vi "Parameters File Handler.vi"(7 "parameters path ctl ref":refnum<vi>, 8 "error in":errorcluster, 10 "selected parameters file":path caption="path to parameters xml", 11 "configuration files page data":T1 {"custom device ref" format="%.0x"}) -> (0 "error out":errorcluster, 3 "configuration files page data out":T1 {"custom device ref" format="%.0x"})   [LabVIEW 2020, in "Ballard ARINC 429 System Explorer.lvlib" / "Implementation.lvlib"]
uses:
  Implementation.lvlib
  Types/Configuration Files Page Data.ctl
  Types/Path Control.ctl
  Types/Browse Button.ctl
  <vilib>/NI VeriStand/Custom Device API/Custom Device Item Ref.ctl
  Import/ARINC 429 Import.lvlib
  Scripting/Ballard/Ballard ARINC 429 Scripting.lvlib
  <vilib>/NI VeriStand/Custom Device API/Custom Device API.lvlib
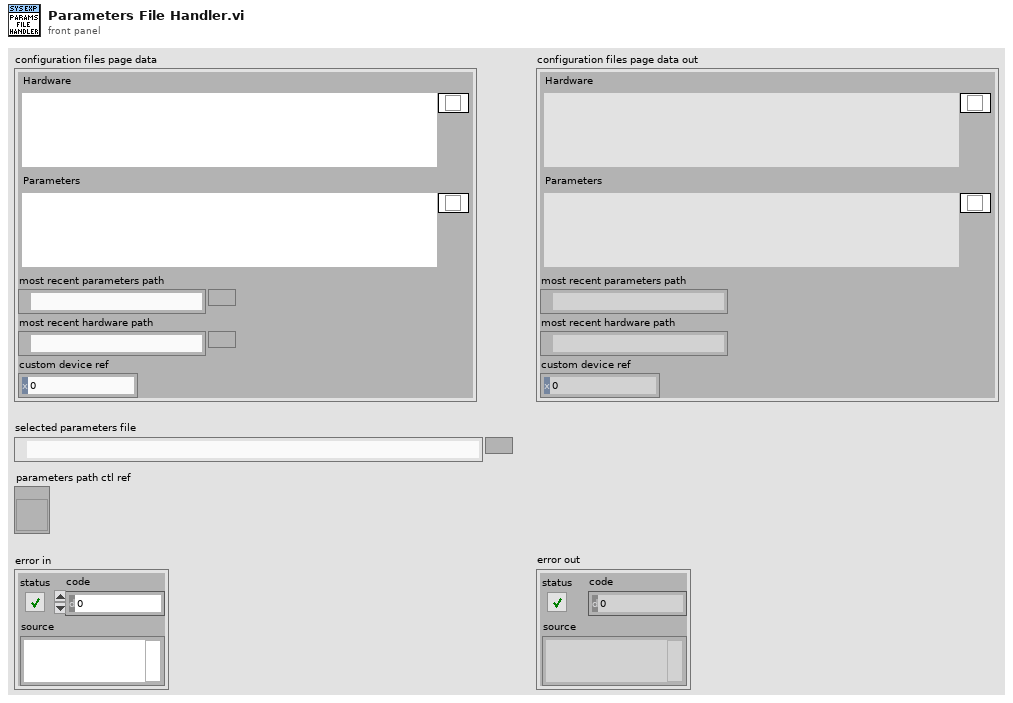
[diagram p1: front panel]
types:
  T1 = typedef "Ballard ARINC 429 System Explorer.lvlib/Implementation.lvlib/Configuration Files Page Data.ctl" = cluster{"Hardware":T2, "Parameters":T2, "most recent parameters path":path, "most recent hardware path":path, "custom device ref":T4}
  T2 = typedef "Ballard ARINC 429 System Explorer.lvlib/Implementation.lvlib/Path Control.ctl" = cluster{"file path":path, "Browse":T3}
  T3 = typedef "Ballard ARINC 429 System Explorer.lvlib/Implementation.lvlib/Browse Button.ctl" = bool
  T4 = typedef "Custom Device API.lvlib/Custom Device Item Ref.ctl" = u64
  T5 = typedef "VS Channels Definition for All Labels on Hardware Channel.ctl" = cluster{"hardware channel":i32, "labels":T6[]}
  T6 = typedef "VS Channels Definition for Label.ctl" = cluster{"label (Dec)":u32, "parameters":T7[], "SDI value":u8, "SDI enabled":bool, "transfer type":T11}
  T7 = typedef "VS Channel Definition for Parameter.ctl" = cluster{"name":string, "direction":T8, "default value":dbl, "unit":string, "Parameter":T9}
  T8 = typedef "Direction.ctl" = enum16{"Rx", "Tx"}
  T9 = typedef "Parameter Definition.ctl" = cluster{"start index":i32, "size":i32, "encoding":T10, "signed":bool, "scale multiplier":dbl, "scale offset":dbl}
  T10 = typedef "Encoding and Decoding.lvlib/Encoding.ctl" = enum16{"BNR", "BCD", "Discrete"}
  T11 = typedef "Transfer Type.ctl" = enum16{"Scheduled", "Acyclic", "Block", "Strobe"}
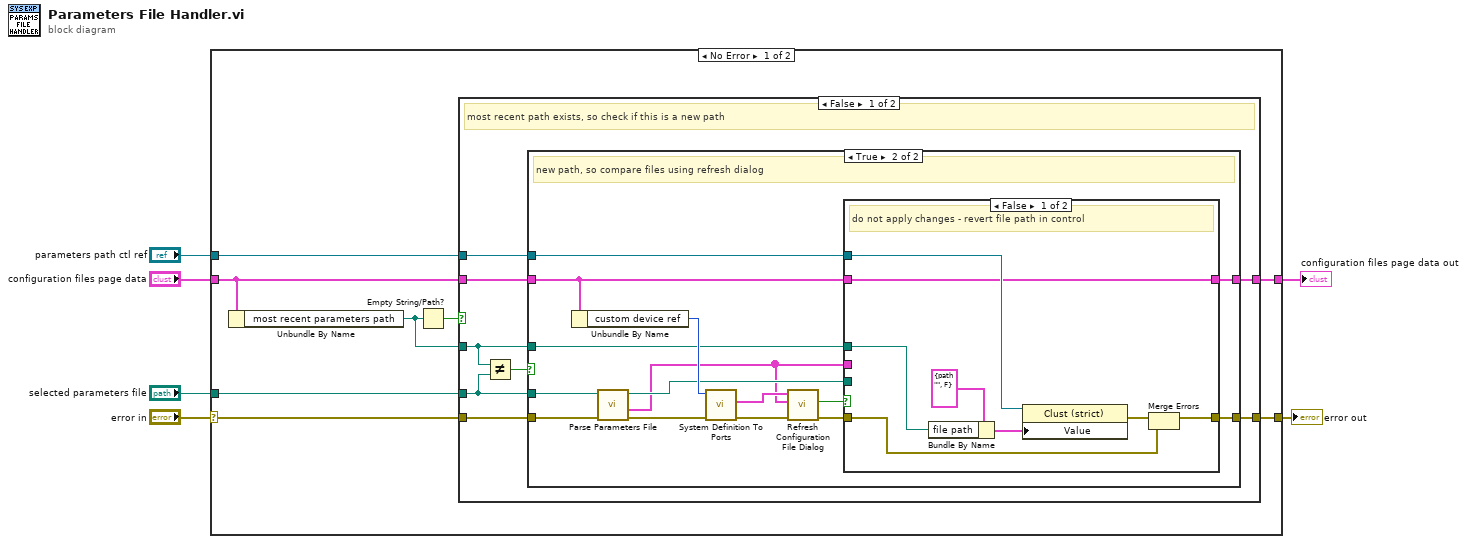
[diagram p0: block diagram]
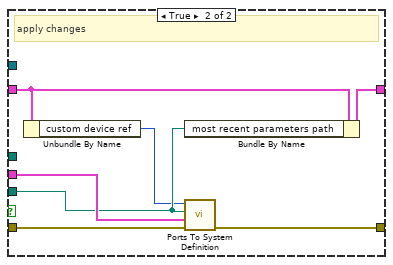
[diagram p3: hidden frame]
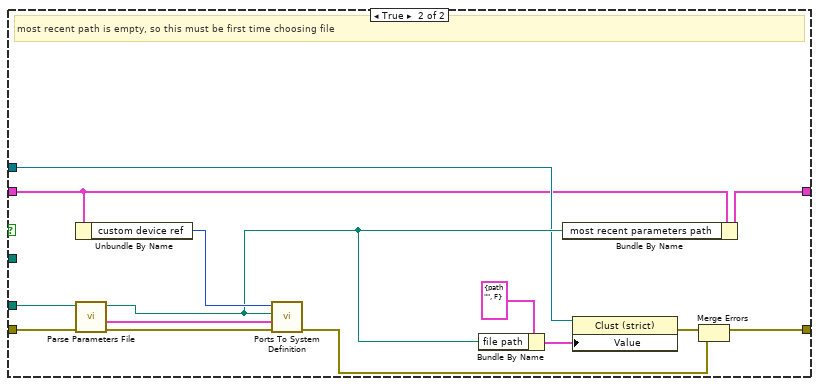
[diagram p4: hidden frame]
diagram:
  n1 = case shown="No Error" "error in" {
    selector: "error in" -> [w14 w70]
    tunnel: [w13 w70] -> w5
    tunnel: "configuration files page data" -> [w11 w69]
    tunnel: [w9 w69] -> w3
    tunnel: "selected parameters file" -> [w12 _]
    tunnel: "parameters path ctl ref" -> [w10 _]
    frame No Error {
      n2 = Unbundle By Name(w11) -> ("most recent parameters path"=w7:path)
      n3 = Empty String/Path?(string/path=w7) -> (empty?=w8:bool)
      n4 = case shown="False" w8 {
        tunnel: w14 -> [w21 w68]
        tunnel: w12 -> [w20 w67]
        tunnel: [w19 w60] -> w13
        tunnel: w7 -> [w18 _]
        tunnel: w11 -> [w17 w56]
        tunnel: w10 -> [w16 w57]
        tunnel: [w15 w55] -> w9
        frame False {
          # "most recent path exists, so check if this is a new path"
          n5 = Not Equal?(x=w18, y=w20) -> (x != y?=w22:bool)
          n6 = case shown="True" w22 {
            tunnel: w21 -> [w24 w39]
            tunnel: w20 -> [_ w28]
            tunnel: [w24 w30] -> w19
            tunnel: w18 -> [_ w29]
            tunnel: w17 -> [w23 w27]
            tunnel: w16 -> [_ w26]
            tunnel: [w23 w25] -> w15
            frame False {
              # "same path, so do nothing"
            }
            frame True {
              # "new path, so compare files using refresh dialog"
              n7 = Unbundle By Name(w27) -> ("custom device ref"=w37:T4)
              n8 = call "Parse Parameters File.vi"("error in"=w39, "path to XML document"=w28) -> ("error out"=w38:errorcluster, "ports"=w31:T5[], "path to XML document out"=w32:path)  [unwired: 7 in]
              n9 = call "System Definition To Ports.vi"("error in"=w38, "custom device ref"=w37) -> ("error out"=w36:errorcluster, "ports"=w35:T5[])  [unwired: 7 in, 1 out]
              n10 = call "Refresh Configuration File Dialog.vi"("error in"=w36, "new ports"=w31, "current ports"=w35) -> ("error out"=w33:errorcluster, "apply changes"=w34:bool)  [unwired: 7 in]
              n11 = case shown="False" w34 {
                tunnel: w33 -> [w42 w54]
                tunnel: w32 -> [_ w52]
                tunnel: w31 -> [_ w53]
                tunnel: [w44 w51] -> w30
                tunnel: w29 -> [w45 _]
                tunnel: w26 -> [w41 _]
                tunnel: w27 -> [w40 w49]
                tunnel: [w40 w50] -> w25
                frame False {
                  # "do not apply changes - revert file path in control"
                  n12 = Bundle By Name(cluster=T2 {"file path"=path "", "Browse"=FALSE} ("Value"), "file path"=w45) -> (w46:T2)
                  n13 = property class="Clust (strict)"(reference=w41, "Value"=w46) -> (error out=w43:errorcluster)  [unwired: 1 in, 1 out]
                  n14 = Merge Errors(w43, w42) -> (w44:errorcluster)
                }
                frame True {
                  # "apply changes"
                  n15 = Unbundle By Name(w49) -> ("custom device ref"=w48:T4)
                  n16 = Bundle By Name(cluster=w49, "most recent parameters path"=w52) -> (w50:T1)
                  n17 = call "Ports To System Definition.vi"("error in"=w54, "ports"=w53, "parameter configuration file path"=w52, "custom device ref"=w48) -> ("error out"=w51:errorcluster)  [unwired: 6 in, 1 out]
                }
              }
            }
          }
        }
        frame True {
          # "most recent path is empty, so this must be first time choosing file"
          n18 = Unbundle By Name(w56) -> ("custom device ref"=w64:T4)
          n19 = call "Parse Parameters File.vi"("error in"=w68, "path to XML document"=w67) -> ("error out"=w66:errorcluster, "ports"=w65:T5[], "path to XML document out"=w58:path)  [unwired: 7 in]
          n20 = call "Ports To System Definition.vi"("error in"=w66, "ports"=w65, "parameter configuration file path"=w58, "custom device ref"=w64) -> ("error out"=w59:errorcluster)  [unwired: 6 in, 1 out]
          n21 = Bundle By Name(cluster=T2 {"file path"=path "", "Browse"=FALSE} ("Value"), "file path"=w58) -> (w63:T2)
          n22 = Bundle By Name(cluster=w56, "most recent parameters path"=w58) -> (w55:T1)
          n23 = property class="Clust (strict)"(reference=w57, "Value"=w63) -> (error out=w61:errorcluster)  [unwired: 1 in, 1 out]
          n24 = Merge Errors(w61, w59) -> (w60:errorcluster)
        }
      }
    }
    frame Error {
    }
  }
  "error out" <- w5
  "configuration files page data out" <- w3
